vi "Renishaw-XL80_SetUpdateAirCompMethod2.vi"(6 "Pressure [Pa]":dbl, 8 "error in (no error)":errorcluster, 9 "Humidity [%]":dbl, 10 "Air Temp [°C]":dbl, 11 "Renishaw-XL80_EMU in":refnum<class "Renishaw-XL80_EMU.lvclass">) -> (0 "error out":errorcluster, 3 "Renishaw-XL80_EMU out":refnum<class "Renishaw-XL80_EMU.lvclass">)   [LabVIEW 2024, in "Renishaw-XL80_EMU.lvclass"]
doc: "This method updates lambda using supplied values for air temperature (oC), air pressure (Pa), and air humidity (%RH).\n\nDefinition\nHRESULTUpdateAirComp2(\n [in] double dAirTemp,\n [in] double dPressure,\n [in] double dHumidity\n);\nParameters\ndAirTemp\nA variable that specifies the air temperature (in oC).\n\ndPressure\nA variable that specifies the air pressure (in Pa).\n\ndHumidity\nA variable that specifies the air humidity (in %RH).\n\nComments\nThis method will return with an HRESULT of E_FAIL if AutoCompensationMode is not set to AUTO_COMPENSATION_OFF. This warns the client that calculating Lambda whilst it is being automatically updated is somewhat pointless.\n\nIf successful this method will return an HRESULT of S_OK."
uses:
  Renishaw-XL80_EMU.lvclass
  Renishaw-XL80_EMU.lvclass/Renishaw-XL80_EMU.ctl
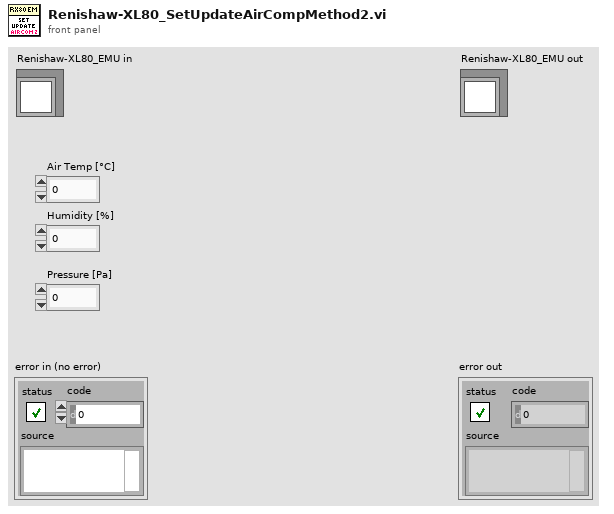
[diagram p1: front panel]
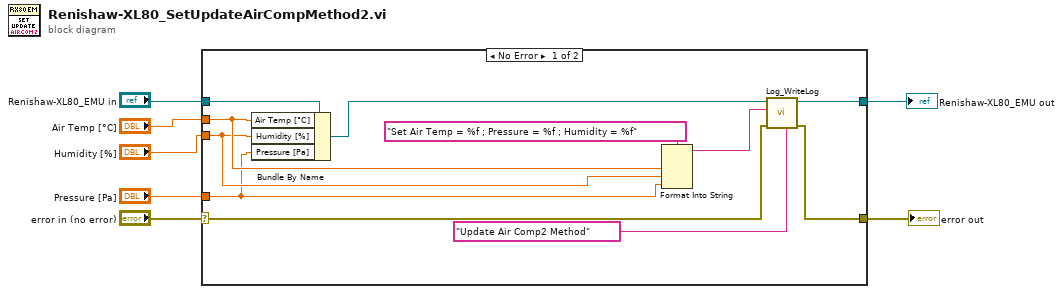
[diagram p0: block diagram]
diagram:
  n1 = case shown="No Error" "error in (no error)" {
    selector: "error in (no error)" -> [w14 w20]
    tunnel: [w13 w20] -> w6
    tunnel: [w15 w19] -> w5
    tunnel: "Renishaw-XL80_EMU in" -> [w18 w19]
    tunnel: "Air Temp [°C]" -> [w10 _]
    tunnel: "Humidity [%]" -> [w9 _]
    tunnel: "Pressure [Pa]" -> [w8 _]
    frame No Error {
      n2 = Bundle By Name(cluster=w18, "Air Temp [°C]"=w10, "Humidity [%]"=w9, "Pressure [Pa]"=w8) -> (w16:refnum<class "Renishaw-XL80_EMU.lvclass">)
      n3 = Format Into String(format string="Set Air Temp = %f ; Pressure = %f ; Humidity = %f", w10, w9, w8) -> (resulting string=w11:string)  [unwired: 2 in, 1 out]
      n4 = call-dynamic "Log_WriteLog.vi"("Additional text"="Update Air Comp2 Method", "error in (no error)"=w14, "Command"=w11, "Log in"=w16) -> ("error out"=w13:errorcluster, "Log out"=w15:refnum<class "Renishaw-XL80_EMU.lvclass">)  [unwired: 6 in]
    }
    frame Error {
    }
  }
  "error out" <- w6
  "Renishaw-XL80_EMU out" <- w5
